vi "FiberSpectrograph_logEvent_measuredSpectrum.vi"(8 "error in (no error)":errorcluster, 11 "logevent_measuredSpectrum_Ctl":T1) -> (0 "error out":errorcluster, 2 "function return":i32, 3 "logevent_measuredSpectrum_Ctl out":T1)   [LabVIEW 2016, in "SALLV_FiberSpectrograph.lvlib"]
doc: "int FiberSpectrograph_shm_logEvent_measuredSpectrumLV(FiberSpectrograph_logevent_measuredSpectrumLV *logevent_measuredSpectrum_Ctl );"
uses:
  SALLV_FiberSpectrograph.lvlib
  DataTypes/logevent_measuredSpectrum.ctl
  SALLV_FiberSpectrograph.so
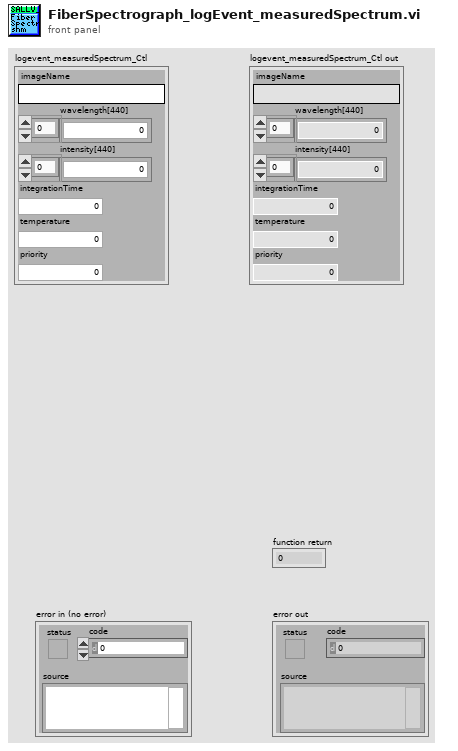
[diagram p1: front panel]
types:
  T1 = typedef "SALLV_FiberSpectrograph.lvlib/logevent_measuredSpectrum.ctl" = cluster{"imageName":string, "wavelength[440]":dbl[], "intensity[440]":dbl[], "integrationTime":sgl, "temperature":dbl, "priority":i32}
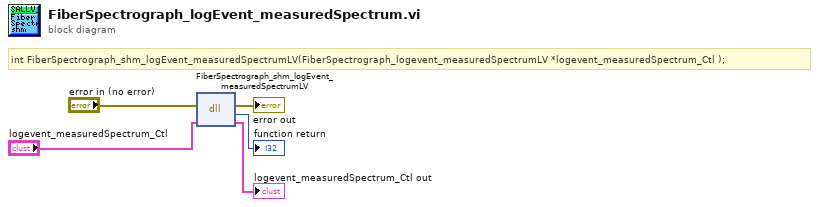
[diagram p0: block diagram]
diagram:
  # "int FiberSpectrograph_shm_logEvent_measuredSpectrumLV(FiberSpectrograph_logevent_measuredSpectrumLV *logevent_measuredSpectrum_Ctl );"
  n1 = dll-call lib="home/harini/tcs/sallv_FiberSpectrometer/SALLV_FiberSpectrograph.*" fn="FiberSpectrograph_shm_logEvent_measuredSpectrumLV"(error in="error in (no error)", "logevent_measuredSpectrum_Ctl"="logevent_measuredSpectrum_Ctl") -> (error out=→"error out":errorcluster, →"function return":i32, "logevent_measuredSpectrum_Ctl"=→"logevent_measuredSpectrum_Ctl out":T1)  [unwired: 2 in, 1 out]
